vi "XY_plot_png.vi"(1 "Job Directory":path=path "/G4_2_HD/Users/paulhayden/Documents/Projects/Hong Roughness/XW data/XW_Corr.tpt") -> (2 "Saved Automatically?":bool, 3 "Tex Info String":string, 4 "Plot data file":path)   [LabVIEW 2018]
uses:
  <vilib>/Analysis/baseanly.llb/Mean (DBL).vi
  Results_plotter_Global.vi
  Data plotting/subVIs/Plot_Values_Global.vi
  <vilib>/Analysis/NI_AALBase.lvlib
panel:
  in  "Black and white":bool
  in  "Blank over":string
  out "Plot Filename":string
  in  "Manual scale?":bool
  out "Current filename index":i32
  in  "Save Automatically?":bool
  in  "Show percentage change?":bool
  out "Table":string[][](table)
  out "XY Graph":cluster{dbl[], dbl[]}[](graph)
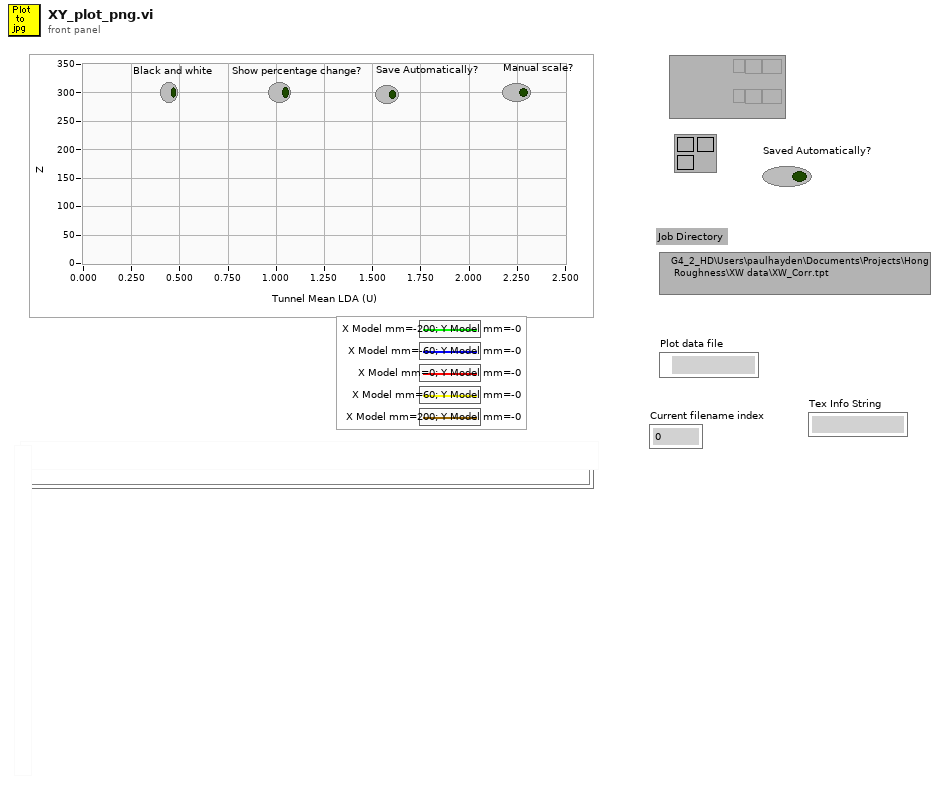
[diagram p1: front panel]
types:
  T1 = typedef "LVRectTypeDef.ctl" = cluster{"Left":i16, "Top":i16, "Right":i16, "Bottom":i16}
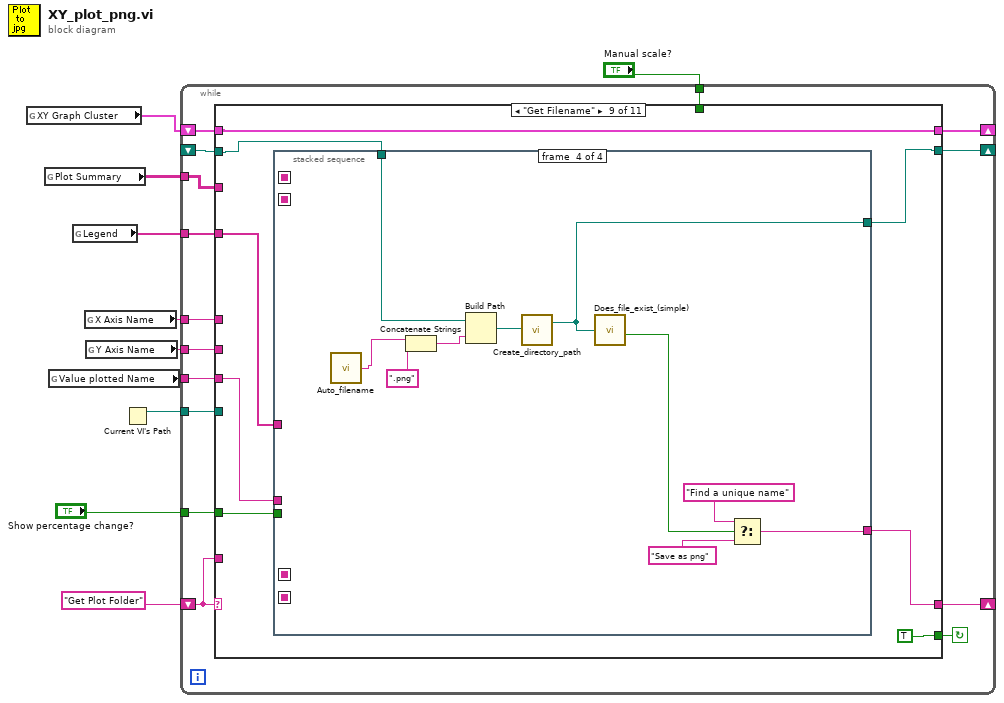
[diagram p0: block diagram]
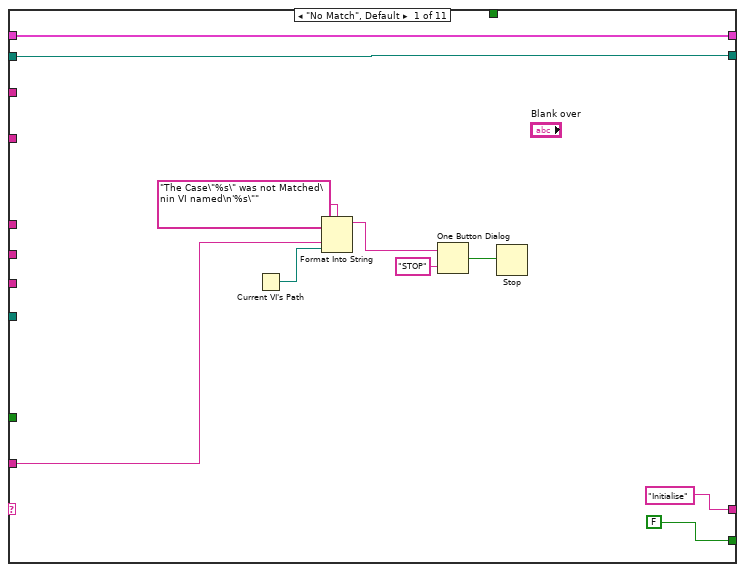
[diagram p2: hidden frame]
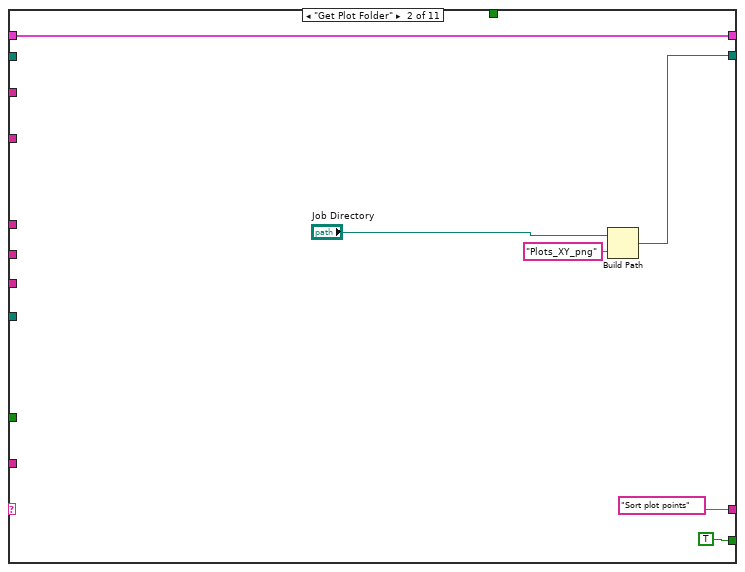
[diagram p3: hidden frame]
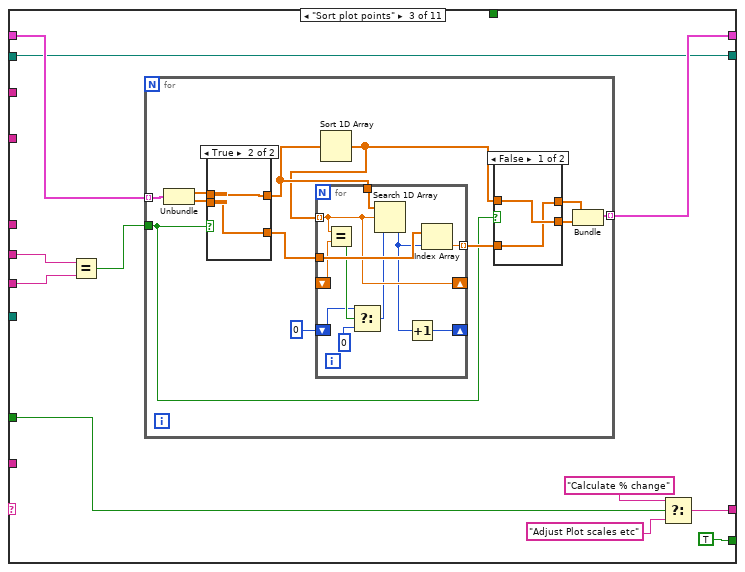
[diagram p4: hidden frame]
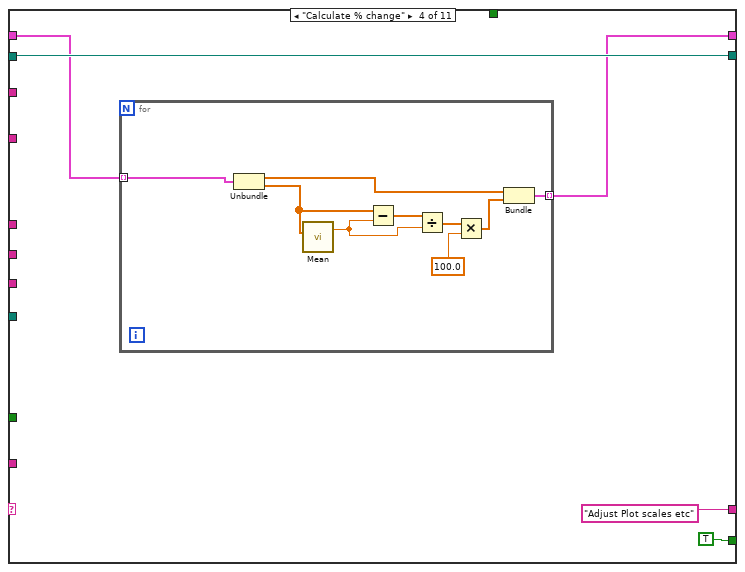
[diagram p7: hidden frame]
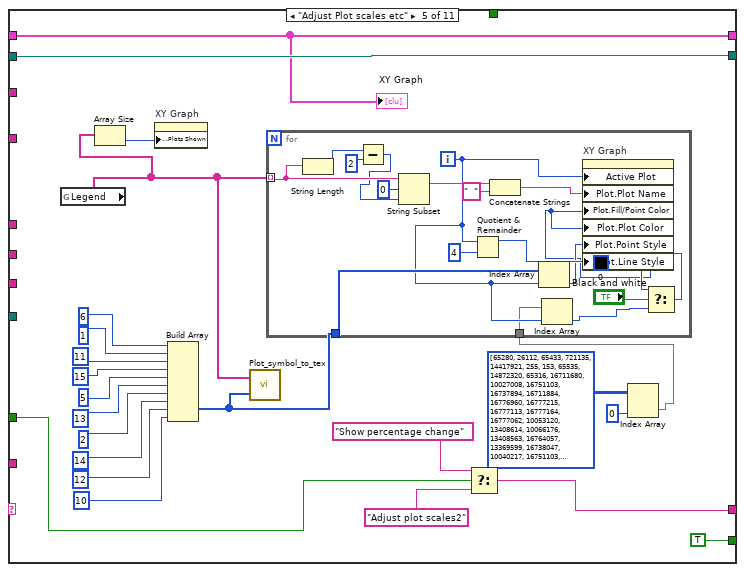
[diagram p8: hidden frame]
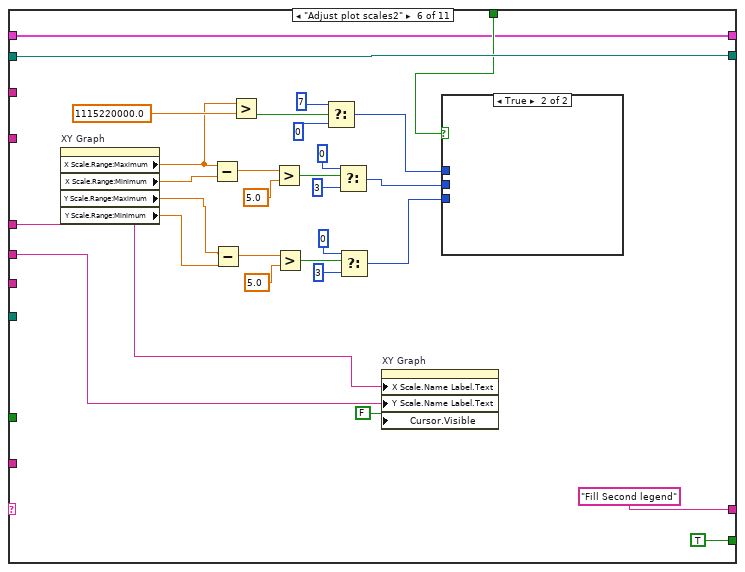
[diagram p9: hidden frame]
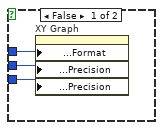
[diagram p10: hidden frame]
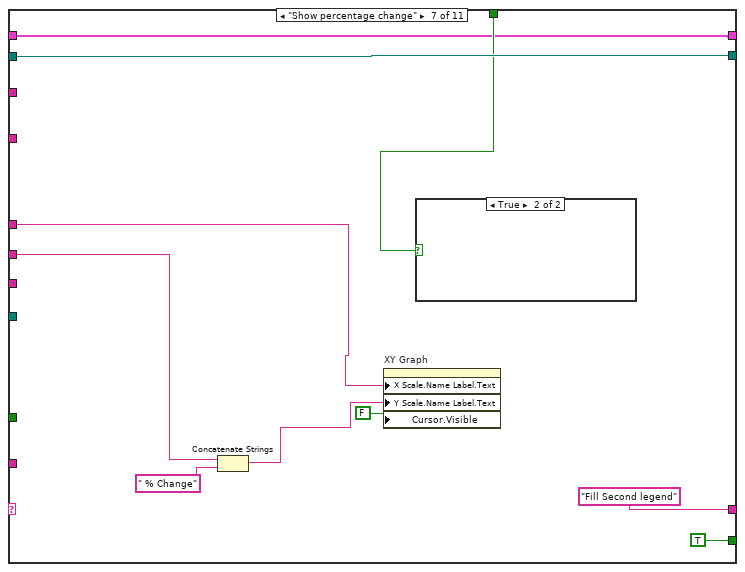
[diagram p11: hidden frame]
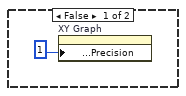
[diagram p12: hidden frame]
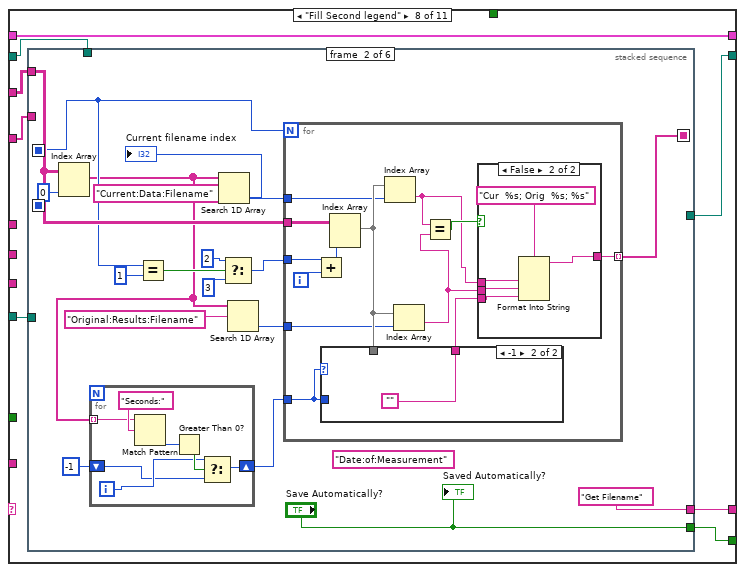
[diagram p13: hidden frame]
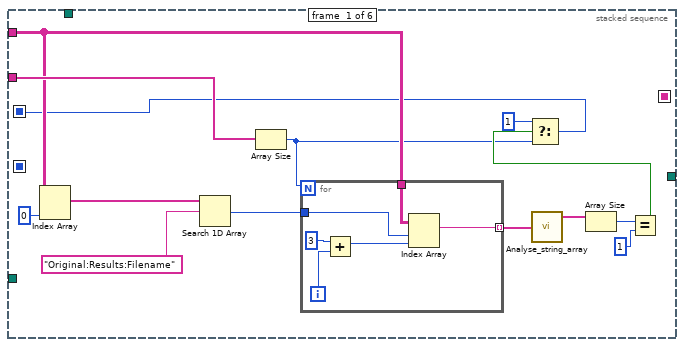
[diagram p14: hidden frame]
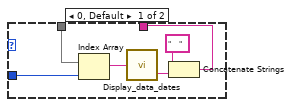
[diagram p15: hidden frame]
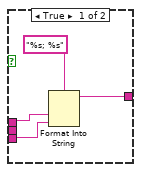
[diagram p16: hidden frame]
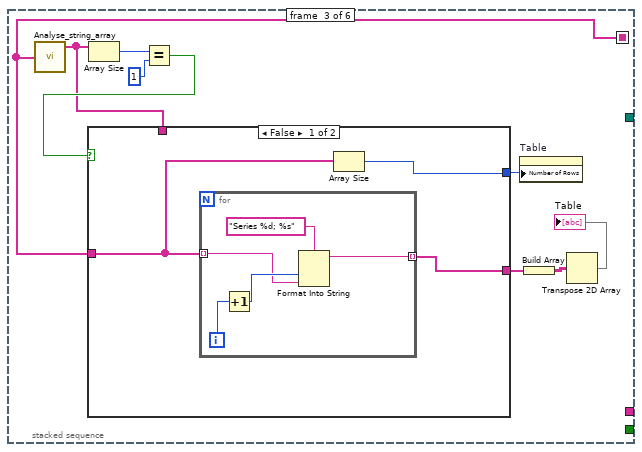
[diagram p17: hidden frame]
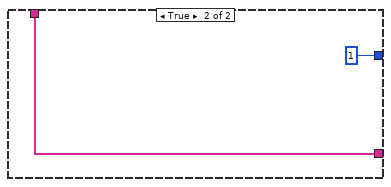
[diagram p18: hidden frame]
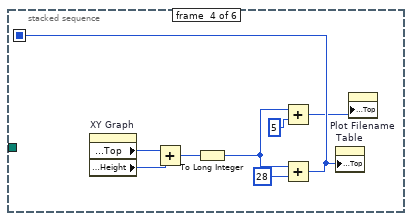
[diagram p19: hidden frame]
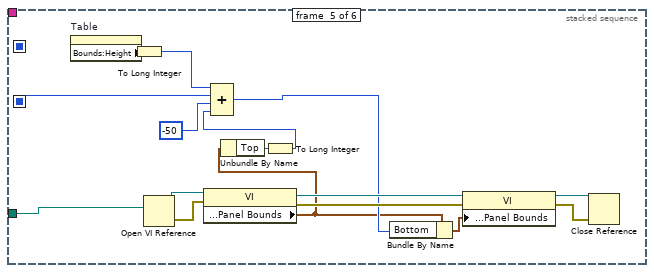
[diagram p20: hidden frame]
diagram:
  n1 = global read "Plot_Values_Global.vi" "XY Graph Cluster"() -> (w1:cluster{dbl[], dbl[]}[])
  n2 = global read "Results_plotter_Global.vi" "Plot Summary"() -> (w8:string[][])
  n3 = global read "Results_plotter_Global.vi" "Value plotted Name"() -> (w4:string)
  n4 = global read "Results_plotter_Global.vi" "Legend"() -> (w7:string[])
  n5 = global read "Results_plotter_Global.vi" "X Axis Name"() -> (w6:string)
  n6 = global read "Results_plotter_Global.vi" "Y Axis Name"() -> (w5:string)
  n7 = Current VI's Path() -> (path=w9:path)
  n8 = while {
    shift-left: "Get Plot Folder" -> [w23]
    shift-right: [w24] -> _
    tunnel: w9 -> [w22]
    tunnel: w8 -> [w21]
    tunnel: w7 -> [w20]
    shift-right: [w19] -> _
    shift-left: _ -> [w18]
    tunnel: "Show percentage change?" -> [w17]
    tunnel: w6 -> [w16]
    tunnel: w5 -> [w15]
    tunnel: w4 -> [w14]
    tunnel: "Manual scale?" -> [w13]
    shift-right: [w11] -> _
    shift-left: w1 -> [w12]
    stop <- w25 continue-if-true
    n9 = case shown="\"Get Filename\"" w23 {
      tunnel: [FALSE TRUE TRUE TRUE TRUE ("Top Level") TRUE ("Top Level") TRUE ("Top Level") w188 TRUE ("Top Level") TRUE ("Top Level") FALSE ("Top Level")] -> w25
      tunnel: ["Initialise" "Sort plot points" w44 "Adjust Plot scales etc" w118 "Fill Second legend" "Fill Second legend" w189 w325 "Save as png" "End"] -> w24
      tunnel: w23 -> [w30 _ _ _ _ _ _ _ _ _ _]
      tunnel: w22 -> [_ _ _ _ _ _ _ w186 _ _ w463]
      tunnel: w21 -> [_ _ _ _ _ _ _ w187 _ _ _]
      tunnel: w20 -> [_ _ _ _ _ _ _ w185 w328 _ _]
      tunnel: [w27 w37 w48 w86 w107 w143 w175 w183 w326 w434 w461] -> w19
      tunnel: w18 -> [w27 _ w48 w86 w107 w143 w175 w184 w327 w435 w461]
      tunnel: w17 -> [_ _ w45 _ w106 _ _ _ w324 _ _]
      tunnel: w16 -> [_ _ _ _ _ w142 w174 _ _ _ _]
      tunnel: w15 -> [_ _ w46 _ _ w141 w173 _ _ _ _]
      tunnel: w14 -> [_ _ w47 _ _ _ _ _ w323 _ _]
      tunnel: w13 -> [_ _ _ _ _ w140 w172 _ _ _ _]
      tunnel: w12 -> [w26 w39 w50 w85 w103 w139 w171 w182 w322 w433 w460]
      tunnel: [w26 w39 w49 w84 w103 w139 w171 w182 w322 w433 w460] -> w11
      frame "No Match", Default {
        n10 = Current VI's Path() -> (path=w29:path)
        n11 = Format Into String(format string="The Case\"%s\" was not Matched\nin VI named\n'%s\"" ("Format String"), w30, w29) -> (resulting string=w33:string)  [unwired: 2 in, 1 out]
        n12 = One Button Dialog(message=w33, button name ("OK")="STOP") -> (true=w31:bool)
        n13 = Stop(stop? (T)=w31) -> ()
      }
      frame "Get Plot Folder" {
        n14 = Build Path(base path="Job Directory", name or relative path="Plots_XY_png") -> (appended path=w37:path)
      }
      frame "Sort plot points" {
        n15 = Equal?(x=w46, y=w47) -> (x = y?=w51:bool)
        n16 = for {
          tunnel: w50 -> [w63] mode=indexing
          tunnel: [w64] -> w49 mode=indexing
          tunnel: w51 -> [w56]
          n17 = Unbundle(w63) -> (w62:dbl[], w59:dbl[])
          n18 = case shown="True" w56 {
            tunnel: [w81 w83] -> w55
            tunnel: w62 -> [w80 w83]
            tunnel: w59 -> [w81 w82]
            tunnel: [w80 w82] -> w58
            frame False {
            }
            frame True {
            }
          }
          n19 = Sort 1D Array(array=w55) -> (sorted array=w54:dbl[])
          n20 = for {
            tunnel: w55 -> [w75]
            tunnel: w54 -> [w71] mode=indexing
            tunnel: w58 -> [w74]
            tunnel: [w73] -> w57 mode=indexing
            shift-right: [w65] -> _
            shift-left: 0 ("f") -> [w68]
            shift-right: [w71] -> _
            shift-left: _ -> [w72]
            n21 = Equal?(x=w71, y=w72) -> (x = y?=w69:bool)
            n22 = Select(t=w68, s=w69, f=0) -> (s? t:f=w66:i32)
            n23 = Search 1D Array(1D array=w75, element=w71, start index (0)=w66) -> (index of element=w70:i32)
            n24 = Increment(x=w70) -> (x+1=w65:i32)
            n25 = Index Array(array=w74, index=w70) -> (element=w73:dbl)
          }
          n26 = case shown="False" w56 {
            tunnel: [w76 w79] -> w61
            tunnel: w54 -> [w77 w79]
            tunnel: [w77 w78] -> w60
            tunnel: w57 -> [w76 w78]
            frame False {
            }
            frame True {
            }
          }
          n27 = Bundle(w61, w60) -> (w64:cluster{dbl[], dbl[]})  [unwired: 1 in]
        }
        n28 = Select(t="Calculate % change", s=w45, f="Adjust Plot scales etc") -> (s? t:f=w44:string)
      }
      frame "Calculate % change" {
        n29 = for {
          tunnel: w85 -> [w97] mode=indexing
          tunnel: [w89] -> w84 mode=indexing
          n30 = Unbundle(w97) -> (w91:dbl[], w96:dbl[])
          n31 = call-poly <vilib>:"Mean.vi"("X"=w96) -> ("mean"=w94:dbl)  [unwired: 1 out]
          n32 = Subtract(x=w96, y=w94) -> (x-y=w95:dbl[])
          n33 = Divide(x=w95, y=w94) -> (x/y=w93:dbl[])
          n34 = Multiply(x=w93, y=100.0) -> (x*y=w90:dbl[])
          n35 = Bundle(w91, w90) -> (w89:cluster{dbl[], dbl[]})  [unwired: 1 in]
        }
      }
      frame "Adjust Plot scales etc" {
        n36 = global read "Results_plotter_Global.vi" "Legend"() -> (w101:string[])
        n37 = Array Size(array=w101) -> (size(s)=w116:i32)
        n38 = property on="XY Graph" class="XYGraph (strict)"("Legend:Plots Shown"=w116) -> ()  [unwired: 2 in, 2 out]
        n39 = Build Array(u8 6 ("Write Attribute"), u8 1 ("Write Attribute"), u8 11 ("Write Attribute"), u8 15 ("Write Attribute"), u8 5 ("Write Attribute"), u8 13 ("Write Attribute"), u8 2 ("Write Attribute"), u8 14 ("Write Attribute"), u8 12 ("Write Attribute"), u8 10 ("Write Attribute")) -> (w102:u8[])
        n40 = call "Plot_symbol_to_tex.vi"("Symbol array"=w102, "Legend"=w101) -> ()  [unwired: 1 out]
        n41 = Select(t="Show percentage change", s=w106, f="Adjust plot scales2") -> (s? t:f=w118:string)
        n42 = Index Array(array=u32[][] [[65280, 26112, 65433, 721135, 14417921], [255, 153, 65535, 14872320, 65316], [16711680, 10027008, 16751103, 16737894, 16711884], [16776960, 16777215, 16777113, 16777164, 16777062], [10053120, 13408614, 10066176, 13408563, 16764057], [13369599, 16738047, 10040217, 16751103, 10040268], [13421772, 5000268, 13421772, 10066329, 16777215], [65535, 6750207, 10092543, 52479, 10092543]] ("Output Array 2"), index (col)=0 ("disabled index (col)")) -> (element=w98:u32[])  [unwired: 1 in]
        n43 = for {
          tunnel: w101 -> [w133] mode=indexing
          tunnel: w102 -> [w136]
          tunnel: w98 -> [w125]
          i -> [w126]
          n44 = String Length(string=w133) -> (length=w129:i32)
          n45 = Subtract(x=w129, y=2) -> (x-y=w127:i32)
          n46 = String Subset(string=w133, offset (0)=0, length (rest)=w127) -> (substring=w132:string)
          n47 = Quotient & Remainder(x=w126, y=4) -> (x-y*floor(x/y)=w137:i32)  [unwired: 1 out]
          n48 = Concatenate Strings(w132, "  " ("string")) -> (w130:string)
          n49 = Index Array(array=w136, index=w126) -> (element=w135:u8)
          n50 = Index Array(array=w125, index=w126) -> (element=w123:u32)
          n51 = Select(t=u32 0, s="Black and white", f=w123) -> (s? t:f=w121:u32)
          n52 = property on="XY Graph" class="XYGraph (strict)"("Active Plot"=w126, "Plot.Plot Name"=w130, "Plot.Fill/Point Color"=w121, "Plot.Plot Color"=w121, "Plot.Point Style"=w135, "Plot.Line Style"=w137) -> ()  [unwired: 2 in, 2 out]
        }
        "XY Graph" <- w103
      }
      frame "Adjust plot scales2" {
        n53 = property on="XY Graph" class="XYGraph (strict)"() -> ("X Scale.Range:Maximum"=w151:dbl, "X Scale.Range:Minimum"=w150:dbl, "Y Scale.Range:Maximum"=w149:dbl, "Y Scale.Range:Minimum"=w148:dbl)  [unwired: 2 in, 2 out]
        n54 = Subtract(x=w151, y=w150) -> (x-y=w153:dbl)
        n55 = Subtract(x=w149, y=w148) -> (x-y=w162:dbl)
        n56 = Greater?(x=w151, y=1115220000.0) -> (0:w165:bool)
        n57 = Greater?(x=w153, y=5.0) -> (0:w155:bool)
        n58 = Greater?(x=w162, y=5.0) -> (0:w160:bool)
        n59 = Select(t=u8 7 ("Write Attribute"), s=w165, f=u8 0 ("Write Attribute")) -> (s? t:f=w147:u8)
        n60 = Select(t=u8 0 ("Write Attribute"), s=w155, f=u8 3) -> (s? t:f=w146:u8)
        n61 = Select(t=u8 0 ("Write Attribute"), s=w160, f=u8 3) -> (s? t:f=w145:u8)
        n62 = property on="XY Graph" class="XYGraph (strict)"("X Scale.Name Label.Text"=w142, "Y Scale.Name Label.Text"=w141, "Cursor.Visible"=FALSE) -> ()  [unwired: 2 in, 2 out]
        n63 = case shown="True" w140 {
          tunnel: w147 -> [w170 _]
          tunnel: w146 -> [w169 _]
          tunnel: w145 -> [w168 _]
          frame False {
            n64 = property on="XY Graph" class="XYGraph (strict)"("X Scale.Format & Precision:Format"=w170, "X Scale.Format & Precision:Precision"=w169, "Y Scale.Format & Precision:Precision"=w168) -> ()  [unwired: 2 in, 2 out]
          }
          frame True {
          }
        }
      }
      frame "Show percentage change" {
        n65 = Concatenate Strings(w173, " % Change" ("string")) -> (w176:string)
        n66 = property on="XY Graph" class="XYGraph (strict)"("X Scale.Name Label.Text"=w174, "Y Scale.Name Label.Text"=w176, "Cursor.Visible"=FALSE) -> ()  [unwired: 2 in, 2 out]
        n67 = case shown="True" w172 {
          frame False {
            n68 = property on="XY Graph" class="XYGraph (strict)"("Y Scale.Format & Precision:Precision"=u8 1) -> ()  [unwired: 2 in, 2 out]
          }
          frame True {
          }
        }
      }
      frame "Fill Second legend" {
        n69 = stacked-sequence {
          seq-local: [_ w220 _ _ _ _] -> [_ _ w264 _ _ _]
          seq-local: [_ _ _ w287 _ _] -> [_ _ _ _ w305 _]
          seq-local: [w190 _ _ _ _ _] -> [_ w219 _ _ _ _]
          tunnel: [_ "Get Filename" _ _ _ _] -> w189
          tunnel: [_ "Save Automatically?" _ _ _ _] -> w188
          tunnel: w187 -> [w194 w221 _ _ _ _]
          tunnel: w186 -> [_ _ _ _ w306 _]
          tunnel: w185 -> [w195 _ _ _ _ _]
          tunnel: w184 -> [_ _ _ _ _ w308]
          tunnel: [_ _ _ _ _ w307] -> w183
          frame #0 {
            n70 = Index Array(array=w194, index (col)=0 ("disabled index (col)")) -> (element=w201:string[])  [unwired: 1 in]
            n71 = Search 1D Array(1D array=w201, element="Original:Results:Filename") -> (index of element=w200:i32)  [unwired: 1 in]
            n72 = Array Size(array=w195) -> (size(s)=w192:i32)
            n73 = for {
              N: w192 -> [_]
              tunnel: w200 -> [w207]
              tunnel: w194 -> [w206]
              tunnel: [w204] -> w196 mode=indexing
              i -> [w209]
              n74 = Add(x=3, y=w209) -> (x+y=w205:i32)
              n75 = Index Array(array=w206, index (row)=w207, index (col)=w205) -> (element=w204:string)
            }
            n76 = call "Analyse_string_array.vi"("String array"=w196) -> ("Unique strings"=w197:string[])  [unwired: 1 in, 1 out]
            n77 = Array Size(array=w197) -> (size(s)=w199:i32)
            n78 = Equal?(x=w199, y=1) -> (x = y?=w193:bool)
            n79 = Select(t=1, s=w193, f=w192) -> (s? t:f=w190:i32)
          }
          frame #1 {
            (unwired) "Date:of:Measurement"
            n80 = Index Array(array=w221, index (col)=0 ("disabled index (col)")) -> (element=w212:string[])  [unwired: 1 in]
            n81 = for {
              tunnel: w212 -> [w233] mode=indexing
              shift-right: [w228] -> w211
              shift-left: -1 -> [w229]
              i -> [w230]
              n82 = Match Pattern(string=w233, regular expression="Seconds:") -> (offset past match=w232:i32)  [unwired: 1 in, 3 out]
              n83 = Greater Than 0?(x=w232) -> (x > 0?=w231:bool)
              n84 = Select(t=w230, s=w231, f=w229) -> (s? t:f=w228:i32)
            }
            n85 = Equal?(x=w219, y=1) -> (x = y?=w217:bool)
            n86 = Search 1D Array(1D array=w212, element="Current:Data:Filename") -> (index of element=w224:i32)  [unwired: 1 in]
            "Current filename index" <- w224
            n87 = Select(t=2, s=w217, f=3 ("disabled index (col)")) -> (s? t:f=w215:i32)
            n88 = Search 1D Array(1D array=w212, element="Original:Results:Filename") -> (index of element=w225:i32)  [unwired: 1 in]
            n89 = for {
              N: w219 -> [_]
              tunnel: w211 -> [w235]
              tunnel: w225 -> [w246]
              tunnel: w224 -> [w245]
              tunnel: w221 -> [w244]
              tunnel: [w242] -> w220 mode=indexing
              tunnel: w215 -> [w238]
              i -> [w241]
              n90 = Add(x=w238, y=w241) -> (x+y=w243:i32)
              n91 = Index Array(array=w244, index (col)=w243) -> (element=w247:string[])  [unwired: 1 in]
              n92 = case shown="-1" w235 {
                tunnel: w247 -> [w253 _]
                tunnel: w235 -> [w252 _]
                tunnel: [w248 ""] -> w236
                frame 0, Default {
                  n93 = Index Array(array=w253, index=w252) -> (element=w251:string)
                  n94 = call "Display_data_dates.vi"("String"=w251) -> ("resulting string"=w250:string)
                  n95 = Concatenate Strings("    " ("string"), w250) -> (w248:string)
                }
                frame -1 {
                }
              }
              n96 = Index Array(array=w247, index=w245) -> (element=w237:string)
              n97 = Index Array(array=w247, index=w246) -> (element=w240:string)
              n98 = Equal?(x=w237, y=w240) -> (x = y?=w239:bool)
              n99 = case shown="False" w239 {
                tunnel: [w257 w262] -> w242
                tunnel: w237 -> [w256 w259]
                tunnel: w240 -> [_ w260]
                tunnel: w236 -> [w255 w261]
                frame True {
                  n100 = Format Into String(format string="%s; %s", w256, w255) -> (resulting string=w257:string)  [unwired: 2 in, 1 out]
                }
                frame False {
                  n101 = Format Into String(format string="Cur  %s; Orig  %s; %s", w259, w260, w261) -> (resulting string=w262:string)  [unwired: 2 in, 1 out]
                }
              }
            }
            "Saved Automatically?" <- "Save Automatically?"
          }
          frame #2 {
            n102 = call "Analyse_string_array.vi"("String array"=w264) -> ("Unique strings"=w267:string[])  [unwired: 1 in, 1 out]
            n103 = Array Size(array=w267) -> (size(s)=w272:i32)
            n104 = Equal?(x=w272, y=1) -> (x = y?=w270:bool)
            n105 = case shown="False" w270 {
              tunnel: w267 -> [_ w282]
              tunnel: [w275 w282] -> w266
              tunnel: [w273 1] -> w265
              tunnel: w264 -> [w274 _]
              frame False {
                n106 = for {
                  tunnel: w274 -> [w278] mode=indexing
                  tunnel: [w276] -> w275 mode=indexing
                  i -> [w280]
                  n107 = Increment(x=w280) -> (x+1=w279:i32)
                  n108 = Format Into String(format string="Series %d; %s", w279, w278) -> (resulting string=w276:string)  [unwired: 2 in, 1 out]
                }
                n109 = Array Size(array=w274) -> (size(s)=w273:i32)
              }
              frame True {
              }
            }
            n110 = property on="Table" class="Tbl (strict)"("Number of Rows"=w265) -> ()  [unwired: 2 in, 2 out]
            n111 = Build Array(w266) -> (w269:string[][])
            n112 = Transpose 2D Array(2D array=w269) -> (transposed array=→"Table":string[][])
          }
          frame #3 {
            n113 = property on="XY Graph" class="XYGraph (strict)"() -> ("Legend:Position:Top"=w290:i32, "Legend:Size:Height"=w286:u32)  [unwired: 2 in, 2 out]
            n114 = Add(x=w290, y=w286) -> (x+y=w289:u32)
            n115 = To Long Integer(number=w289) -> (32bit integer=w285:i32)
            n116 = Add(x=w285, y=5) -> (x+y=w283:i32)
            n117 = Add(x=w285, y=28) -> (x+y=w287:i32)
            n118 = property on="Table" class="Tbl (strict)"("Position:Top"=w287) -> ()  [unwired: 2 in, 2 out]
            n119 = property on="Plot Filename" class="Str"("Position:Top"=w283) -> ()  [unwired: 2 in, 2 out]
          }
          frame #4 {
            n120 = property on="Table" class="Tbl (strict)"() -> ("Bounds:Height"=w300:u32)  [unwired: 2 in, 2 out]
            n121 = To Long Integer(number=w300) -> (32bit integer=w295:i32)
            n122 = Open VI Reference(vi path=w306) -> (vi reference=w304:refnum<vi>, error out=w303:errorcluster)  [unwired: 5 in]
            n123 = property class="VI"(reference=w304, error in=w303) -> (reference out=w302:refnum<vi>, error out=w301:errorcluster, "Front Panel Window:Panel Bounds"=w297:T1)
            n124 = Unbundle By Name(w297) -> ("Top"=w296:i16)
            n125 = To Long Integer(number=w296) -> (32bit integer=w294:i32)
            n126 = Compound Arithmetic op=ADD(w295, w305, -50 ("value"), w294) -> (w299:i32)
            n127 = Bundle By Name(cluster=w297, "Bottom"=w299) -> (w293:T1)
            n128 = property class="VI"(reference=w302, error in=w301, "Front Panel Window:Panel Bounds"=w293) -> (reference out=w292:refnum<vi>, error out=w291:errorcluster)
            n129 = Close Reference(reference=w292, error in (no error)=w291) -> ()  [unwired: 1 out]
          }
          frame #5 {
            n130 = global read "Results_plotter_Global.vi" "Current Data Filenames"() -> (w319:string)
            n131 = call "Fast_string_Replace.vi"("Replace match with:"="_", "Input String"=w319, "regular expression"="[/]") -> ("Output String"=w315:string)  [unwired: 1 in, 1 out]
            n132 = call "Fast_string_Replace.vi"("Replace match with:"="_", "Input String"=w315, "regular expression"="__") -> ("Output String"=w318:string)  [unwired: 1 in, 1 out]
            n133 = call "Fast_string_Replace.vi"("Replace match with:"="", "Input String"=w318, "regular expression"=" ") -> ("Output String"=w320:string)  [unwired: 1 in, 1 out]
            n134 = String Subset(string=w320, offset (0)=0, length (rest)=30 ("length (rest)")) -> (substring=w321:string)
            n135 = Build Path(base path=w308, name or relative path=w321) -> (appended path=w307:path)
          }
        }
      }
      frame "Get Filename" {
        n136 = stacked-sequence {
          seq-local: [_ w349 _ _] -> [_ _ w394 _]
          seq-local: [w337 _ _ _] -> [_ w350 _ _]
          seq-local: [w331 _ _ _] -> [_ _ w387 _]
          seq-local: [_ _ w382 _] -> [_ _ _ _]
          tunnel: w328 -> [w340 _ _ _]
          tunnel: w327 -> [_ _ _ w431]
          tunnel: [_ _ _ w430] -> w326
          tunnel: [_ _ _ w426] -> w325
          tunnel: w324 -> [w330 _ _ _]
          tunnel: w323 -> [w334 _ _ _]
          frame #0 {
            n137 = for {
              tunnel: w340 -> [w348] mode=indexing
              shift-right: [w346] -> w338
              shift-left: string[] [] ("String array") -> [w347]
              n138 = call "Get_array_values_fr_String.vi"("String Value"=w348) -> ("String array"=w345:string[])  [unwired: 1 out]
              n139 = Build Array (concatenate)(w347, w345) -> (w346:string[])
            }
            n140 = Match Pattern(string=w334, regular expression="[/]") -> (before substring=w335:string)  [unwired: 1 in, 3 out]
            n141 = case shown="True" w330 {
              tunnel: [w341 w343] -> w333
              tunnel: w335 -> [w341 w344]
              frame False {
              }
              frame True {
                n142 = Concatenate Strings("%" ("string"), w344) -> (w343:string)
              }
            }
            n143 = call "Analyse_string_array.vi"("String array"=w338) -> ("Unique strings"=w337:string[])  [unwired: 1 in, 1 out]
            n144 = Concatenate Strings(w333, "_" ("string")) -> (w331:string)
          }
          frame #1 {
            n145 = for {
              tunnel: w350 -> [w352] mode=indexing
              tunnel: [w351] -> w349 mode=indexing
              n146 = Match Pattern(string=w352, regular expression="[.]") -> (offset past match=w353:i32)  [unwired: 1 in, 3 out]
              n147 = case shown="0, Default" w353 {
                tunnel: [w356 w381] -> w351
                tunnel: w352 -> [w360 w381]
                frame 0, Default {
                  n148 = while {
                    shift-right: [w379] -> _
                    shift-left: w360 -> [w374]
                    tunnel: [w375] -> w359
                    tunnel: [w374] -> w355
                    i -> [w375]
                    stop <- w378 stop-if-true
                    n149 = Decimal Digit?(1:w374) -> (0:w377:bool)
                    n150 = Empty String/Path?(string/path=w374) -> (empty?=w376:bool)
                    n151 = Or(x=w377, y=w376) -> (x .or. y?=w378:bool)
                    n152 = String Subset(string=w374, offset (0)=1) -> (substring=w379:string)  [unwired: 1 in]
                  }
                  n153 = Fract/Exp String To Number(string=w355) -> (offset past number=w357:i32, number=w358:dbl)  [unwired: 3 in]
                  n154 = Greater?(x=w358, y=2.1) -> (0:w361:bool)
                  n155 = case shown="True" w361 {
                    tunnel: w360 -> [w363 w372]
                    tunnel: w359 -> [_ w371]
                    tunnel: w358 -> [_ w370]
                    tunnel: w357 -> [_ w369]
                    tunnel: w355 -> [_ w368]
                    tunnel: [w363 w364] -> w356
                    frame False {
                    }
                    frame True {
                      n156 = Number To Decimal String(number=w370) -> (decimal integer string=w366:string)  [unwired: 1 in]
                      n157 = String Subset(string=w372, offset (0)=0, length (rest)=w371) -> (substring=w367:string)
                      n158 = String Subset(string=w368, offset (0)=w369) -> (substring=w365:string)  [unwired: 1 in]
                      n159 = Concatenate Strings(w367, w366, w365) -> (w364:string)
                    }
                  }
                }
                frame -1 {
                }
              }
            }
          }
          frame #2 {
            n160 = Array Size(array=w394) -> (size(s)=w393:i32)
            n161 = String Length(string=w387) -> (length=w395:i32)
            n162 = Decrement(x=w393) -> (x-1=w392:i32)
            n163 = while {
              tunnel: w394 -> [w403] mode=indexing
              shift-right: [w411] -> _
              shift-left: w395 -> [w413]
              tunnel: w392 -> [w412]
              tunnel: [w406] -> w391
              tunnel: [w405] -> w390
              tunnel: [w404] -> w388 mode=indexing
              i -> [w405]
              stop <- w408 continue-if-true
              n164 = Less?(x=w405, y=w412) -> (x < y?=w407:bool)
              n165 = call "Fast_string_Replace.vi"("Replace match with:"="", "Input String"=w403, "regular expression"="\\[mm]") -> ("Output String"=w418:string)  [unwired: 1 in, 1 out]
              n166 = call "Fast_string_Replace.vi"("Replace match with:"="", "Input String"=w418, "regular expression"=" ") -> ("Output String"=w416:string)  [unwired: 1 in, 1 out]
              n167 = call "Fast_string_Replace.vi"("Replace match with:"="-", "Input String"=w416, "regular expression"="[.]") -> ("Output String"=w404:string)  [unwired: 1 in, 1 out]
              n168 = String Length(string=w404) -> (length=w414:i32)
              n169 = Increment(x=w414) -> (x+1=w409:i32)
              n170 = Add(x=w409, y=w413) -> (x+y=w411:i32)
              n171 = Less?(x=w411, y=26 ("length (rest)")) -> (x < y?=w406:bool)
              n172 = Compound Arithmetic op=AND(w406, w407) -> (w408:bool)
            }
            n173 = case shown="False" w391 {
              tunnel: [w400 w401] -> w389
              tunnel: w390 -> [w400 w402]
              frame False {
              }
              frame True {
                n174 = Increment(x=w402) -> (x+1=w401:i32)
              }
            }
            n175 = for {
              N: w389 -> [_]
              shift-right: [w396] -> w385
              shift-left: w387 -> [w399]
              tunnel: w388 -> [w398] mode=indexing
              n176 = Concatenate Strings(w399, w398, "_" ("string")) -> (w396:string)
            }
            n177 = String Length(string=w385) -> (length=w386:i32)
            n178 = Decrement(x=w386) -> (x-1=w383:i32)
            n179 = String Subset(string=w385, offset (0)=0, length (rest)=w383) -> (substring=w382:string)
          }
          frame #3 {
            n180 = call "Auto_filename.vi"() -> ("Filename"=w425:string)  [unwired: 2 in]
            n181 = Concatenate Strings(w425, ".png" ("string")) -> (w423:string)
            n182 = Build Path(base path=w431, name or relative path=w423) -> (appended path=w432:path)
            n183 = call "Create_directory_path.vi"("Path name"=w432) -> ("Path name Out"=w430:path)  [unwired: 2 in, 1 out]
            n184 = call "Does_file_exist_(simple).vi"("Pathname"=w430) -> ("exists?"=w428:bool)
            n185 = Select(t="Find a unique name", s=w428, f="Save as png") -> (s? t:f=w426:string)
          }
        }
      }
      frame "Find a unique name" {
        w436 = ".png" ("regular expression")
        n186 = Strip Path(path=w435) -> (stripped path=w439:path, name=w440:string)
        n187 = Match Pattern(string=w440, regular expression=w436) -> (before substring=w438:string)  [unwired: 1 in, 3 out]
        n188 = while {
          tunnel: w438 -> [w459]
          tunnel: 27 ("Max Length") -> [w458]
          tunnel: w439 -> [w457]
          tunnel: w436 -> [w456]
          tunnel: [w443] -> w434
          i -> [w445]
          stop <- w444 continue-if-true
          n189 = Add(x=97, y=w445) -> (x+y=w454:i32)
          n190 = Build Array(w454) -> (w455:i32[])
          n191 = Byte Array To String(unsigned byte array=w455) -> (string=w452:string)
          n192 = Concatenate Strings(w459, w452) -> (w450:string)
          n193 = Reverse String(1:w450) -> (0:w451:string)
          n194 = String Subset(string=w451, offset (0)=0, length (rest)=w458) -> (substring=w449:string)
          n195 = Reverse String(1:w449) -> (0:w447:string)
          n196 = Concatenate Strings(w447, w456) -> (w446:string)
          n197 = Build Path(base path=w457, name or relative path=w446) -> (appended path=w443:path)
          n198 = call "Does_file_exist_(simple).vi"("Pathname"=w443) -> ("exists?"=w444:bool)
        }
      }
      frame "Save as png" {
        n199 = stacked-sequence {
          tunnel: w463 -> [_ w486 _]
          tunnel: w461 -> [w473 w478 w503]
          frame #0 {
            w465 = FALSE ("Visible")
            n200 = Path to Array of Strings(0:w473) -> (2:w469:string[])  [unwired: 1 out]
            n201 = Array Size(array=w469) -> (size(s)=w472:i32)
            n202 = property on="Show percentage change?" class="Bool (strict)"("Visible"=w465) -> ()  [unwired: 2 in, 2 out]
            n203 = property on="Black and white" class="Bool (strict)"("Visible"=w465) -> ()  [unwired: 2 in, 2 out]
            n204 = property on="Save Automatically?" class="Bool (strict)"("Visible"=w465) -> ()  [unwired: 2 in, 2 out]
            n205 = Subtract(x=w472, y=3) -> (x-y=w470:i32)
            n206 = Array Subset(array=w469, index=w470) -> (w467:string[])  [unwired: 1 in]
            n207 = for {
              shift-right: [w474] -> w466
              shift-left: "Plot Filename  " ("string") -> [w477]
              tunnel: w467 -> [w475] mode=indexing
              n208 = Concatenate Strings(w477, " :  ", w475) -> (w474:string)
            }
            "Plot Filename" <- w466
            n209 = property on="Manual scale?" class="Bool (strict)"("Visible"=w465) -> ()  [unwired: 2 in, 2 out]
          }
          frame #1 {
            w480 = 8 ("image depth")
            n210 = Open VI Reference(vi path=w486) -> (vi reference=w488:refnum<vi>, error out=w487:errorcluster)  [unwired: 5 in]
            n211 = invoke class="VI" method="FP.Old Get Image"(reference=w488, error in=w487, "visible area only"=TRUE, "image depth"=w480) -> (error out=w484:errorcluster, "image"=w483:u8[], "colors"=w481:u32[], "bounds"=w482:T1)  [unwired: 4 in, 4 out]
            n212 = call <vilib>:"Write PNG File(6_1).vi"("color table"=w481, "depth"=w480, "error in (no error)"=w484, "flattened image data"=w483, "rect"=w482, "path to PNG file"=w478) -> ("error out"=w479:errorcluster)  [unwired: 4 in, 1 out]
            n213 = call <vilib>:"General Error Handler.vi"("error in (no error)"=w479) -> ()  [unwired: 10 in, 5 out]
          }
          frame #2 {
            w490 = TRUE ("Visible")
            n214 = property on="Show percentage change?" class="Bool (strict)"("Visible"=w490) -> ()  [unwired: 2 in, 2 out]
            n215 = property on="Manual scale?" class="Bool (strict)"("Visible"=w490) -> ()  [unwired: 2 in, 2 out]
            n216 = property on="Black and white" class="Bool (strict)"("Visible"=w490) -> ()  [unwired: 2 in, 2 out]
            n217 = property on="Save Automatically?" class="Bool (strict)"("Visible"=w490) -> ()  [unwired: 2 in, 2 out]
            n218 = Strip Path(path=w503) -> (stripped path=w501:path, name=w498:string)
            n219 = String Length(string=w498) -> (length=w500:i32)
            n220 = Build Path(base path=w501, name or relative path="Plot_Data") -> (appended path=w493:path)
            n221 = Subtract(x=w500, y=3) -> (x-y=w496:i32)
            n222 = String Subset(string=w498, offset (0)=0, length (rest)=w496) -> (substring=w495:string)
            n223 = Concatenate Strings(w495, "xls" ("string")) -> (w492:string)
            n224 = Build Path(base path=w493, name or relative path=w492) -> (appended path=w491:path)
            n225 = call "Create_directory_path.vi"("Path name"=w491) -> ("Path name Out"=w489:path)  [unwired: 2 in, 1 out]
            "Plot data file" <- w489
            n226 = call "Delete_with_Check.vi"("FilePath"=w489) -> ()  [unwired: 1 out]
          }
        }
      }
    }
  }
